vi "Remove JSON Tag.vi"(11 "Name":string) -> (2 "tagged as JSON text":bool, 3 "Name (tag stripped)":string)   [LabVIEW 2020, in "Library Commun.lvlib" / "JSON support.lvlib"]
uses:
  support/JSON support.lvlib
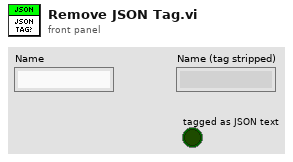
[diagram p1: front panel]
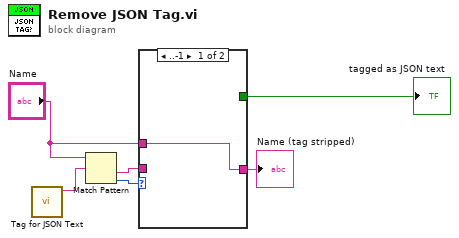
[diagram p0: block diagram]
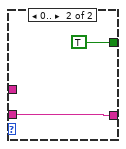
[diagram p2: hidden frame]
diagram:
  n1 = call "Tag for JSON Text.vi"() -> ("Tag for JSON text"=w3:string)  [unwired: 11 in]
  n2 = Match Pattern(string="Name", regular expression=w3) -> (after substring=w4:string, offset past match=w5:i32)  [unwired: 1 in, 2 out]
  n3 = case shown="..-1" w5 {
    tunnel: [w7 w8] -> w1
    tunnel: "Name" -> [w7 _]
    tunnel: w4 -> [_ w8]
    tunnel: [_ TRUE] -> w6
    frame ..-1 {
    }
    frame 0.. {
    }
  }
  "tagged as JSON text" <- w6
  "Name (tag stripped)" <- w1
